vi "TagDB-Release.vi"(8 "error in (no error)":errorcluster, 9 "force destroy? (F)":bool, 11 "TagDB":refnum<k1>) -> (0 "error out":errorcluster)   [LabVIEW 2017, in "TagDB.lvlib"]
uses:
  TagDB.lvlib
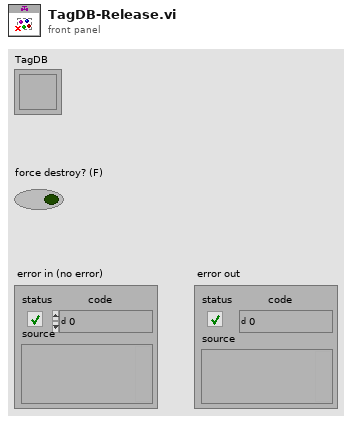
[diagram p1: front panel]
types:
  T1 = enum16{"create", "destroy", "cleanUp", "list", "get info", "force destroy"}
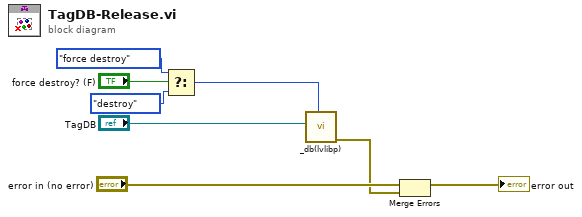
[diagram p0: block diagram]
diagram:
  n1 = Select(t=T1."force destroy" ("command"), s="force destroy? (F)", f=T1."destroy" ("command")) -> (s? t:f=w1:T1)
  n2 = call "_db(lvlibp).vi"("command"=w1, "db in"="TagDB") -> ("error out"=w5:errorcluster)  [unwired: 5 in, 4 out]
  n3 = Merge Errors("error in (no error)", w5) -> (→"error out":errorcluster)
